vi "Client Example.vi"() -> ()   [LabVIEW 2016]
uses:
  <vilib>/rajsite/i3-json/JSON Generation/Create Value Files/Create Value - 1D Array Double.vi
  Classes/Server/Format Client Request (Auto-Increment).vi
  <vilib>/httpClient/POSTBuffer.vi
  <vilib>/httpClient/LabVIEWHTTPClient.lvlib
  Classes/Server/JSONRPC Server.lvclass
  <vilib>/rajsite/i3-json/i3-json.lvlib
panel:
  in  "stop":bool
  out "Response String":string
  in  "Send Sync Request":bool
  in  "A":dbl
  in  "B":dbl
  # "Subtraction"
  # "Synchronous Request"
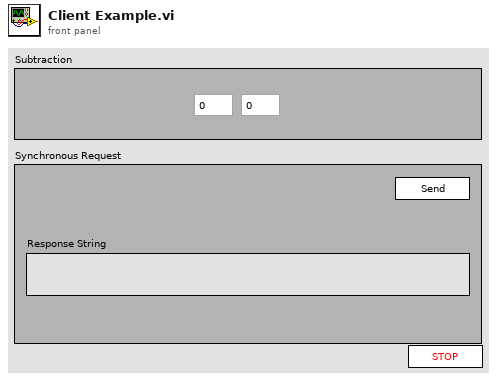
[diagram p1: front panel]
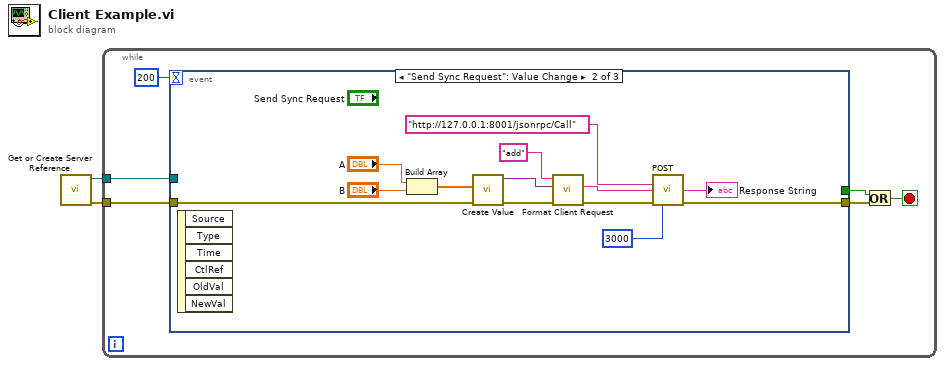
[diagram p0: block diagram]
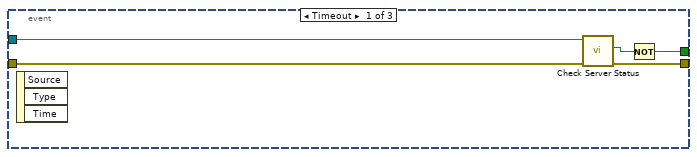
[diagram p2: hidden frame]
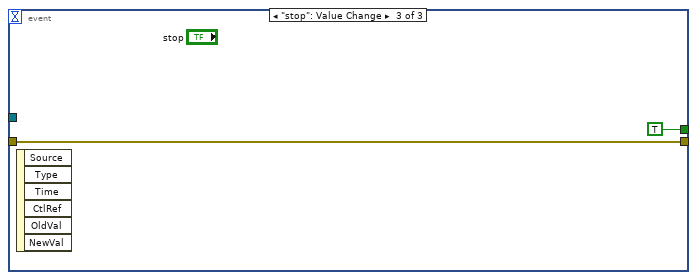
[diagram p3: hidden frame]
diagram:
  n1 = call "Get or Create Server Reference.vi"() -> ("error out"=w1:errorcluster, "Server Out"=w2:refnum<class "JSONRPC Server.lvclass">)  [unwired: 10 in]
  n2 = while {
    tunnel: w2 -> [w8]
    tunnel: w1 -> [w7]
    stop <- w3 stop-if-true
    n3 = event shown="[1] \"Send Sync Request\": Value Change" {
      selector: _ -> [_ _ _]
      dyn-events: _ -> [_ _ _]
      timeout: 200 -> [_ _ _]
      tunnel: w8 -> [w13 _ _]
      tunnel: [w10 _ TRUE] -> w5
      tunnel: [w9 w15 w27] -> w4
      tunnel: w7 -> [w12 w22 w27]
      event Timeout {
        n4 = event-data() -> ()  [unwired: 1 in, 3 out]
        n5 = call "Check Server Status.vi"("error in (no error)"=w12, "Request in"=w13) -> ("error out"=w9:errorcluster, "Server Running?"=w11:bool)  [unwired: 7 in, 1 out]
        n6 = Not(x=w11) -> (.not. x?=w10:bool)
      }
      event "Send Sync Request": Value Change {
        n7 = event-data() -> ()  [unwired: 1 in, 6 out]
        n8 = Build Array("A", "B") -> (w25:dbl[])
        n9 = call-poly <vilib>:"Create Value.vi"("error in (no error)"=w22, "1D Numeric"=w25) -> ("error out"=w23:errorcluster, "JSON Tree"=w24:variant)  [unwired: 8 in]
        n10 = call-poly "Format Client Request.vi"("error in (no error)"=w23, "params"=w24, "method"="add") -> ("error out"=w16:errorcluster, "Request String"=w20:string)  [unwired: 7 in]
        n11 = call-poly <vilib>:"POST.vi"("url"="http://127.0.0.1:8001/jsonrpc/Call", "buffer"=w20, "error in (no error)"=w16, "timeout (10000)"=3000) -> ("body"=→"Response String":string, "error out"=w15:errorcluster)  [unwired: 8 in, 2 out]
      }
      event "stop": Value Change {
        n12 = event-data() -> ()  [unwired: 1 in, 6 out]
      }
    }
    n13 = Or(x=w5, y=w4) -> (x .or. y?=w3:bool)
  }
